vi "test-632.vi"(8 "error in (no error)":errorcluster, 11 "TestCase in":refnum<class "testcase-issue.lvclass">) -> (0 "error out":errorcluster, 3 "TestCase out":refnum<class "testcase-issue.lvclass">)   [LabVIEW 2017, in "testcase-issue.lvclass"]
uses:
  testcase-issue.lvclass
  <vilib>/addons/_JKI Toolkits/VI Tester/TestCase.llb/TestCase.lvclass
  C:/Program Files (x86)/National Instruments/LabVIEW 2017/vi.lib/addons/_JKI Toolkits/VI Tester/TestCase.llb/TestCase.lvclass
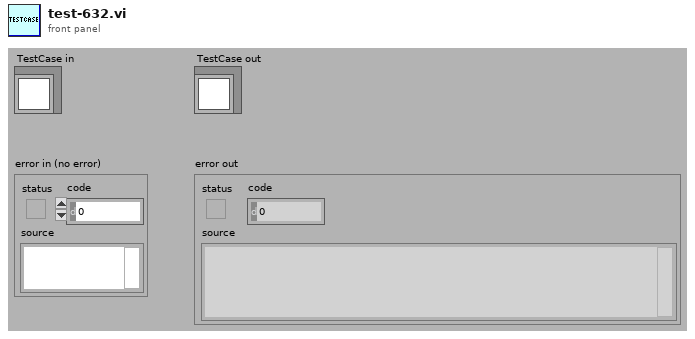
[diagram p1: front panel]
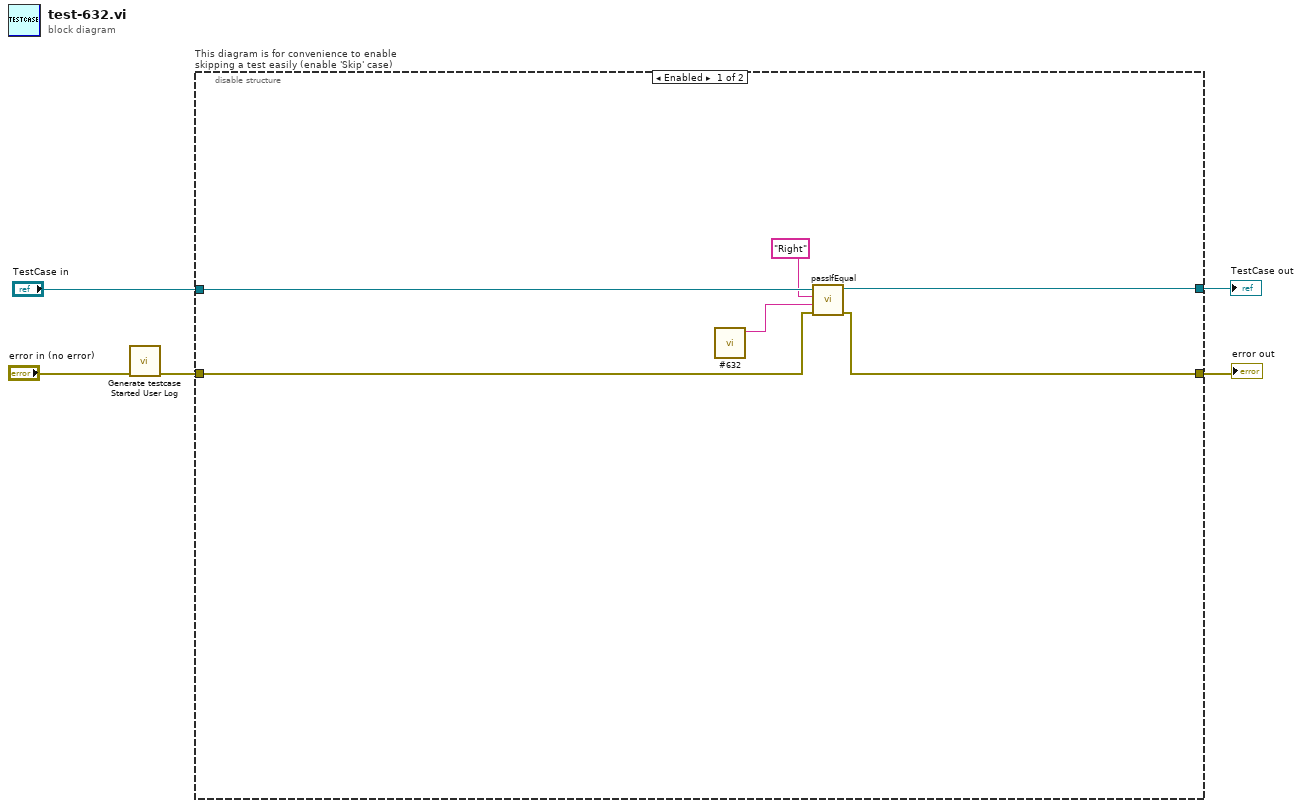
[diagram p0: block diagram]
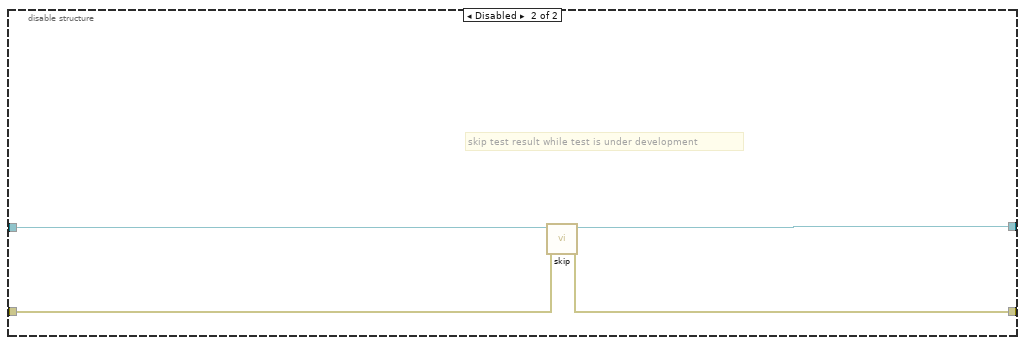
[diagram p2: hidden frame]
diagram:
  n1 = call "Generate testcase Started User Log.vi"("Error In"="error in (no error)") -> ("error out"=w1:errorcluster)  [unwired: 10 in]
  n2 = disable-structure "This diagram is for convenience to enable skipping a test easily (enable 'Skip' case)" shown="Enabled" {
    disable-tunnel: "TestCase in" -> [w9 w15]
    disable-tunnel: [w11 w13] -> w2
    disable-tunnel: [w10 w14] -> w4
    disable-tunnel: w1 -> [w8 w12]
    frame Enabled {
      n3 = call "#632.vi"() -> ("Arguments"=w7:string)  [unwired: 11 in]
      n4 = call-dynamic "passIfEqual.vi"("error in (no error)"=w8, "y"=w7, "x"="Right" ("Arguments"), "TestCase in"=w9) -> ("error out"=w10:errorcluster, "TestCase out"=w11:refnum<class "testcase-issue.lvclass">)  [unwired: 6 in]
    }
    frame Disabled {
      # "skip test result while test is under development"
      n5 = call <vilib>:"skip.vi"("error in (no error)"=w12, "TestCase in"=w15) -> ("error out"=w14:errorcluster, "TestCase out"=w13:refnum<class "testcase-issue.lvclass">)  [unwired: 8 in]
    }
  }
  "error out" <- w4
  "TestCase out" <- w2
